vi "getBroadcastData.vi"   [LabVIEW 2013, in "EC1000-control.lvlib" / "SM1000-control.lvclass"]
doc: "Get embedded controller device data.\n\nThis function is used by a client application to retrieve various types of data related to the specified EC1000 module."
uses:
  SM1000-control.lvclass
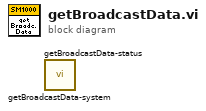
[diagram p0: block diagram]
diagram:
  n1 = call "getBroadcastData-system.vi"() -> ()  [unwired: 9 in, 3 out]
  n2 = call "getBroadcastData-status.vi"() -> ()  [unwired: 9 in, 3 out]
